vi "matrix_filter - forvard.vi"(0 "field":T1, 1 "matrix in":dbl[][](array[numeric])=array1x4097[4097 elements], 5 "intensity/phase":i16(ring) items=["int", "pha"], 9 "multiplication/substitution":i16(ring) items=["subst", "mult"], 11 "error in (no error)":errorcluster, 12 "forward distance":dbl) -> (4 "field out":T1, 15 "error out":errorcluster)   [LabVIEW 2012, in "Lightpipes.lvlib"]
uses:
  LightPipes.lvlib
panel:
  out "number of columns":i32
  out "number of rows":i32
  out "matrix 1D":dbl[](array[numeric])
  out "matrix out":dbl[](array[numeric])
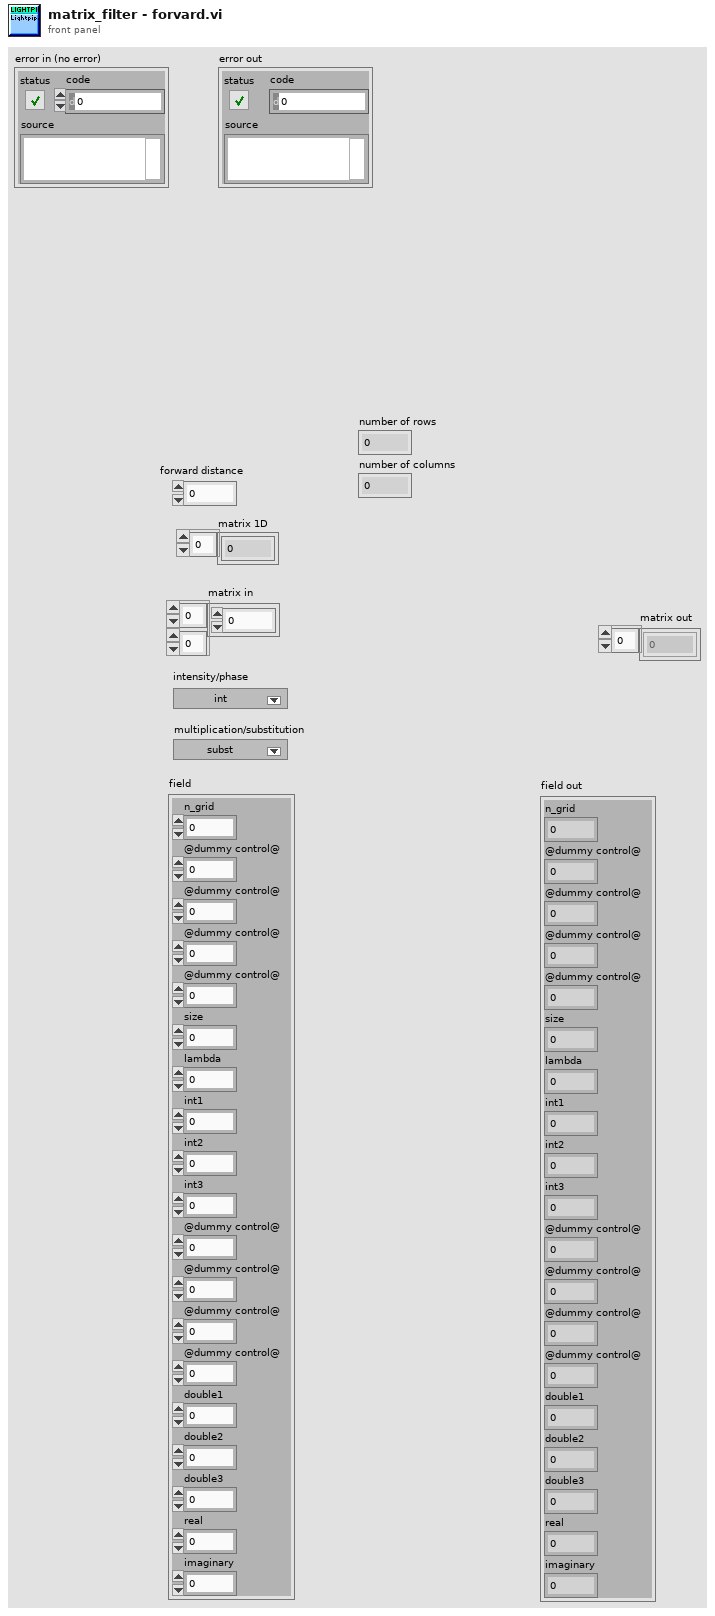
[diagram p1: front panel]
types:
  T1 = cluster{"n_grid":i32, "@dummy control@":i8, "@dummy control@":i8, "@dummy control@":i8, "@dummy control@":i8, "size":dbl, "lambda":dbl, "int1":i32, "int2":i32, "int3":i32, "@dummy control@":i8, "@dummy control@":i8, "@dummy control@":i8, "@dummy control@":i8, "double1":dbl, "double2":dbl, "double3":dbl, "real":u32, "imaginary":u32}
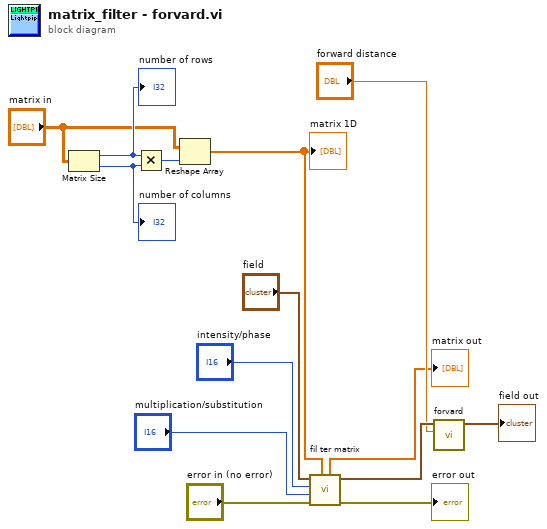
[diagram p0: block diagram]
diagram:
  n1 = Matrix Size(0:"matrix in") -> (1:w6:i32, 2:w5:i32)
  "number of rows" <- w6
  "number of columns" <- w5
  n2 = Multiply(x=w6, y=w5) -> (x*y=w3:i32)
  n3 = Reshape Array "Reshape Array"("matrix in", w3) -> (w7:dbl[])
  "matrix 1D" <- w7
  n4 = call "fil ter matrix.vi"("matrix"=w7, "error in (no error)"="error in (no error)", "multiplication/ substitution"="multiplication/substitution", "intensity / phase"="intensity/phase", "field"="field") -> ("error out"=→"error out":errorcluster, "field out"=w13:T1, "matrix out"=→"matrix out":dbl[])  [unwired: 4 in]
  n5 = call "forvard.vi"("distance"="forward distance", "field"=w13) -> ("field out"=→"field out":T1)  [unwired: 9 in]
